vi "Single SSC DCPower Export Signal.vi"(0 "DCPower SSC in":T2, 5 "signal":T1=1030 items=["Source Complete Event"=1030, "Measure Complete Event"=1031, "Sequence Iteration Complete Event"=1032, "Sequence Engine Done Event"=1033, "Pulse Complete Event"=1051, "Ready For Pulse Trigger Event"=1052, "Start Trigger"=1034, "Source Trigger"=1035, "Measure Trigger"=1036, "Sequence Advance Trigger"=1037, "Pulse Trigger"=1053], 7 "output terminal":tag, 11 "error in":errorcluster) -> (4 "DCPower SSC out":T2, 15 "error out":errorcluster)   [LabVIEW 2020]
doc: "Routes signals (triggers and events) to the output terminal you specify for a session."
uses:
  SSC DCPower.ctl
  <instrlib>/niDCPower/nidcpower.llb/niDCPower Export Signal - Signal.ctl
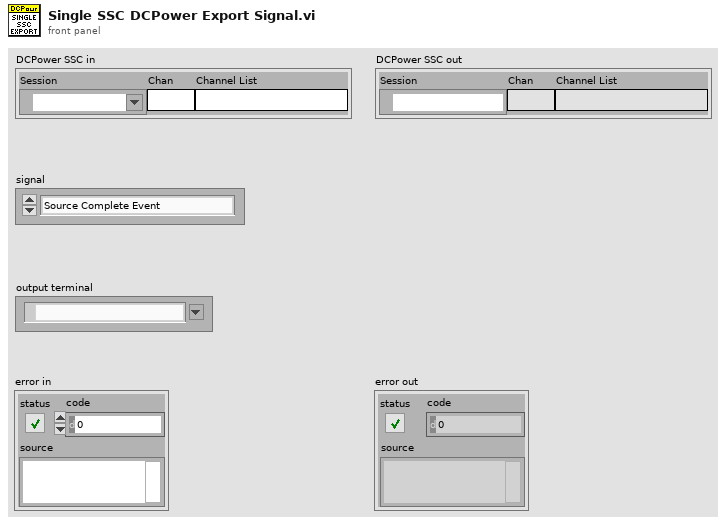
[diagram p1: front panel]
types:
  T1 = typedef "niDCPower Export Signal - Signal.ctl" = i32
  T2 = typedef "SSC DCPower.ctl" = cluster{"Session":refnum<k15>, "Chan":string, "Channel List":string}
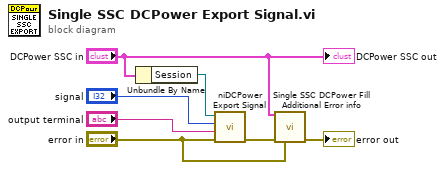
[diagram p0: block diagram]
diagram:
  n1 = Unbundle By Name("DCPower SSC in") -> ("Session"=w4:refnum<k15>)
  n2 = call <instrlib>:"niDCPower Export Signal.vi"("error in (no error)"="error in", "output terminal"="output terminal", "signal"="signal", "instrument handle"=w4) -> ("error out"=w5:errorcluster)  [unwired: 6 in, 1 out]
  n3 = call "Single SSC DCPower Fill Additional Error info.vi"("DCPower SSC in"="DCPower SSC in", "error in"=w5, "previous error in"="error in") -> ("error out"=→"error out":errorcluster)  [unwired: 12 in]
  "DCPower SSC out" <- "DCPower SSC in"
